vi "Read Device List State from File.vi"(8 "Error In":errorcluster, 10 "file":path, 11 "Device List State":T1) -> (0 "Error Out":errorcluster, 2 "file out":path, 3 "Device List State out":T1)   [LabVIEW 2015]
uses:
  Device List State.ctl
  Device/Device.lvclass
  Dynamic FP XControl/Name type and data.ctl
  Device/Device type.ctl
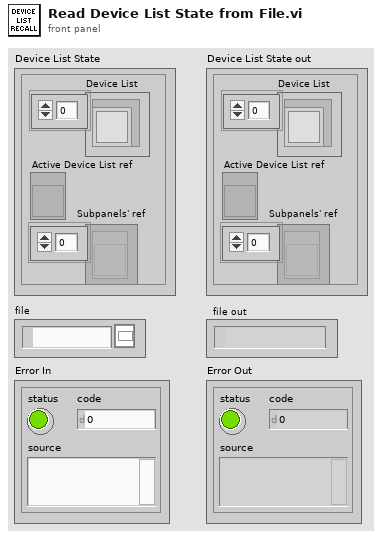
[diagram p1: front panel]
types:
  T1 = typedef "Device List State.ctl" = cluster{"Device List":refnum<class "Device.lvclass">[], "Active Device List ref":refnum<vi>, "Subpanels' ref":refnum<vi>[]}
  T2 = enum16{"open", "open or create", "create or replace", "create", "open (read-only)"}
  T3 = typedef "Name type and data.ctl" = cluster{"Front Panel Data":variant, "Device type":T4, "Name":string}
  T4 = typedef "Device type.ctl" = enum16{"NONE", "Neocera 21", "LakeShore 335", "LakeShore 340", "LkShr 340 chA&B", "LakeShore 370", "SRS 850", "SRS 830", "LR 700", "EG&G 5302", "EG&G 7260", "EG&G 7280", "AH 2500", "Keithley meter", "Keithley electrometer", "Keithley 182", "HP 5385", "HP 53181", "HP 53132", "ITC503", "IPS120", "Oxford Mercury IPS", "Oxford PS", "Test", "DC Facility Magnet", "Cryomagnetics PS", "Keithley 2400", "Keithley current source", "Cryo-Con 22C", "HP87NN", "HP4395A"}
  T5 = cluster{"Saved device":i32, "Present device":i32}[]
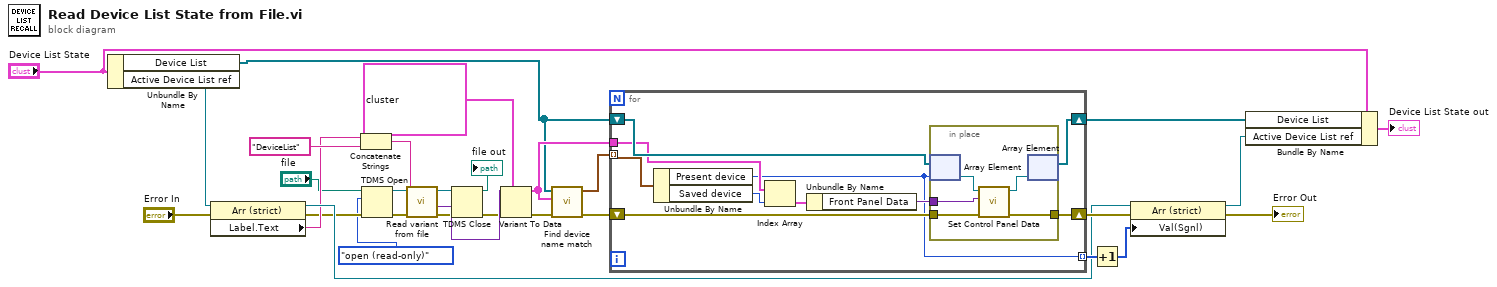
[diagram p0: block diagram]
diagram:
  n1 = Unbundle By Name("Device List State") -> ("Device List"=w21:refnum<class "Device.lvclass">[], "Active Device List ref"=w12:refnum<vi>)
  n2 = property class="Arr (strict)"(reference=w12, error in="Error In") -> (reference out=w13:refnum<vi>, error out=w7:errorcluster, "Label.Text"=w11:string)
  n3 = Concatenate Strings(w11, "DeviceList" ("string")) -> (w29:string)
  n4 = TDMS Open(8:w7, 10:T2."open (read-only)" ("operation (0:open)"), 11:"file") -> (0:w8:errorcluster, 3:w4:refnum<k34>)  [unwired: 4 in]
  n5 = call "Read variant from file.vi"("error in (no error)"=w8, "group name in"=w29, "tdms file"=w4) -> ("error out"=w26:errorcluster, "variant out"=w28:variant, "tdms file out"=w2:refnum<k34>)  [unwired: 6 in]
  n6 = TDMS Close(8:w26, 11:w2) -> (0:w3:errorcluster, 3:→"file out":path)
  n7 = Variant To Data(error in=w3, type=T3[] [{"Front Panel Data"=variant, "Device type"=enum."NONE", "Name"=""}], Variant=w28) -> (data=w23:T3[], error out=w25:errorcluster)
  n8 = call "Find device name match.vi"("error in"=w25, "Saved names and data"=w23, "Device list"=w21) -> ("error out"=w22:errorcluster, "Matching pairs"=w24:T5)  [unwired: 7 in]
  n9 = for {
    tunnel: w24 -> [w39] mode=indexing
    shift-right: [w37] -> w19
    shift-left: w21 -> [w40]
    tunnel: w23 -> [w38]
    shift-right: [w34] -> w18
    shift-left: w22 -> [w35]
    tunnel: [w31] -> w16 mode=indexing
    n10 = Unbundle By Name(w39) -> ("Present device"=w31:i32, "Saved device"=w32:i32)
    n11 = Index Array(array=w38, index=w32) -> (element=w36:T3)
    n12 = Unbundle By Name(w36) -> ("Front Panel Data"=w33:variant)
    n13 = in-place {
      in-place-border: w33 -> [w43]
      in-place-border: w35 -> [w42]
      in-place-border: [w41] -> w34
      n14 = in-place-array #1(w40, w31) -> (w45:refnum<class "Device.lvclass">)
      n15 = call "Set Control Panel Data.vi"("error in (no error)"=w42, "Data"=w43, "Device in"=w45) -> ("error out"=w41:errorcluster, "Device out"=w44:refnum<class "Device.lvclass">)  [unwired: 7 in]
      n16 = in-place-array #1(w44) -> (w37:refnum<class "Device.lvclass">[])  [unwired: 1 out]
    }
  }
  n17 = Increment(x=w16) -> (x+1=w15:i32[])
  n18 = property class="Arr (strict)"(reference=w13, error in=w18, "Val(Sgnl)"=w15) -> (reference out=w17:refnum<vi>, error out=→"Error Out":errorcluster)
  n19 = Bundle By Name(cluster="Device List State", "Device List"=w19, "Active Device List ref"=w17) -> (→"Device List State out":T1)
